vi "GD_MG_MagicFormula_OnOff.vi"(5 "Aktion":enum16{"lesen", "schreiben", "init"}(ring), 7 "use old LNI":bool, 10 "MG_use_magic_formula":bool=TRUE) -> (0 "use old LNI":bool, 3 "MG_use_magic_formula":bool=TRUE)   [LabVIEW 2020, in "Linearisierung v2.lvlib" / "Gasteiler.lvlib"]
uses:
  Gasteiler.lvlib
  Aktionen FGV Gasteiler Daten.ctl
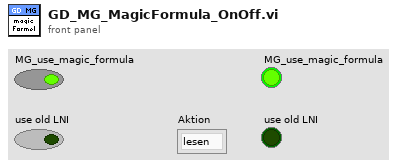
[diagram p1: front panel]
types:
  T1 = typedef "Linearisierung v2.lvlib/Gasteiler.lvlib/Aktionen FGV Gasteiler Daten.ctl" = enum16{"lesen", "Gasteiler Daten", "Seriellen Param.", "MB-Endwert", "laden", "speichern", "Anforderung", "TCP", "Aufzeichnung Start"}
  T2 = typedef "Linearisierung v2.lvlib/Gasteiler.lvlib/Gasteiler Daten.ctl" = cluster{"Gasteiler":T3, "Gasteiler Stufen":T4, "Gasteiler Type":T5, "Konfig Gasteiler":T6, "Gasteiler Span Eingänge":u16}
  T3 = typedef "String - Eingabefeld.ctl" = string
  T4 = typedef "Linearisierung v2.lvlib/Gasteiler.lvlib/Gasteiler Stufen.ctl" = u16
  T5 = typedef "Linearisierung v2.lvlib/GasteilerType.ctl" = u16
  T6 = typedef "System Einstellungen V2.lvlib/Gasteiler Auswahl.ctl" = u16
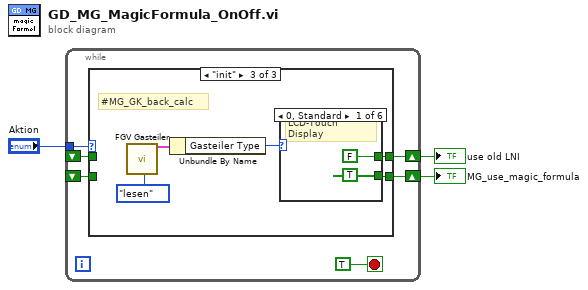
[diagram p0: block diagram]
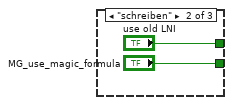
[diagram p3: hidden frame]
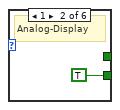
[diagram p4: hidden frame]
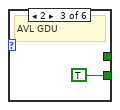
[diagram p5: hidden frame]
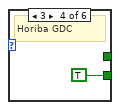
[diagram p6: hidden frame]
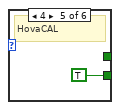
[diagram p7: hidden frame]
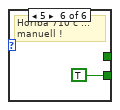
[diagram p8: hidden frame]
diagram:
  n1 = while {
    tunnel: "Aktion" -> [w6]
    shift-right: [w8] -> w2
    shift-left: _ -> [w5]
    shift-right: [w9] -> w3
    shift-left: _ -> [w4]
    stop <- TRUE stop-if-true
    n2 = case shown="\"init\"" w6 {
      tunnel: [w10 "MG_use_magic_formula" w15] -> w9
      tunnel: [w11 "use old LNI" w14] -> w8
      tunnel: w5 -> [w11 _ _]
      tunnel: w4 -> [w10 _ _]
      frame "lesen", Default {
      }
      frame "schreiben" {
      }
      frame "init" {
        # "#MG_GK_back_calc"
        n3 = call "FGV Gasteiler.vi"("Aktionen"=Aktionen_FGV_Gasteiler_Daten."lesen") -> ("Gasteiler Daten"=w17:T2)  [unwired: 11 in, 7 out]
        n4 = Unbundle By Name(w17) -> ("Gasteiler Type"=w16:T5)
        n5 = case shown="0, Standard" w16 {
          tunnel: [TRUE TRUE TRUE TRUE TRUE TRUE] -> w15
          tunnel: [FALSE _ _ _ _ _] -> w14
          frame 0, Default {
            # "LCD-Touch Display"
          }
          frame 1 {
            # "Analog-Display"
          }
          frame 2 {
            # "AVL GDU"
          }
          frame 3 {
            # "Horiba GDC"
          }
          frame 4 {
            # "HovaCAL"
          }
          frame 5 {
            # "Horiba 710 c ... manuell !"
          }
        }
      }
    }
  }
  "MG_use_magic_formula" <- w3
  "use old LNI" <- w2
